vi "Definition and Attributes.vi"(11 "Type in":refnum<class "Type.lvclass">) -> (1 "Attributes":T1, 2 "Definition":T2, 3 "Type out":refnum<class "Type.lvclass">)   [LabVIEW 2020, in "Conditum.lvlib" / "Columns.lvlib" / "Type.lvclass"]
uses:
  Type.lvclass
  Type.lvclass/Type.ctl
  Definition.ctl
  Attributes.ctl
  Conditum.lvlib
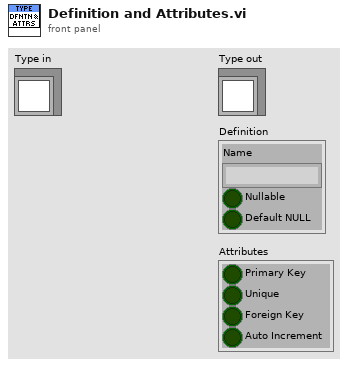
[diagram p1: front panel]
types:
  T1 = typedef "Conditum.lvlib/Attributes.ctl" = cluster{"Primary Key":bool, "Unique":bool, "Foreign Key":bool, "Auto Increment":bool}
  T2 = typedef "Conditum.lvlib/Columns.lvlib/Type.lvclass/Definition.ctl" = cluster{"Name":string, "Nullable":bool, "Default NULL":bool}
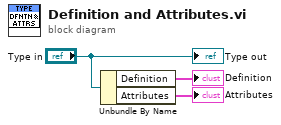
[diagram p0: block diagram]
diagram:
  n1 = Unbundle By Name("Type in") -> ("Definition"=→"Definition":T2, "Attributes"=→"Attributes":T1)
  "Type out" <- "Type in"
